vi "ReadGPS.vi"() -> ()   [LabVIEW 2010]
panel:
  in  "stop":bool
  out "GPS Data":T1 {"Course over ground (degrees)" format="%#.6g"; "Speed over ground (knots)" format="%#.6g"; "Magnetic Variation (degrees)" format="%#.6g"; "Longitude (ddmm.mmmm)" format="%#.6g"; "Lattitude (ddmm.mmmm)" format="%#.6g"}
  out "XY Graph":cluster{"Y":dbl[], "Y":dbl[]}[](graph)
  out "Course over ground (degrees)":dbl(knob) scale=0.0..360.0
  out "Speed over ground (knots)":dbl(knob) scale=0.0..5.0
  out "GPS Data Valid?":bool
  out "error out":errorcluster
  in  "VISA resource name":refnum<visa-resource-name>="COM1"
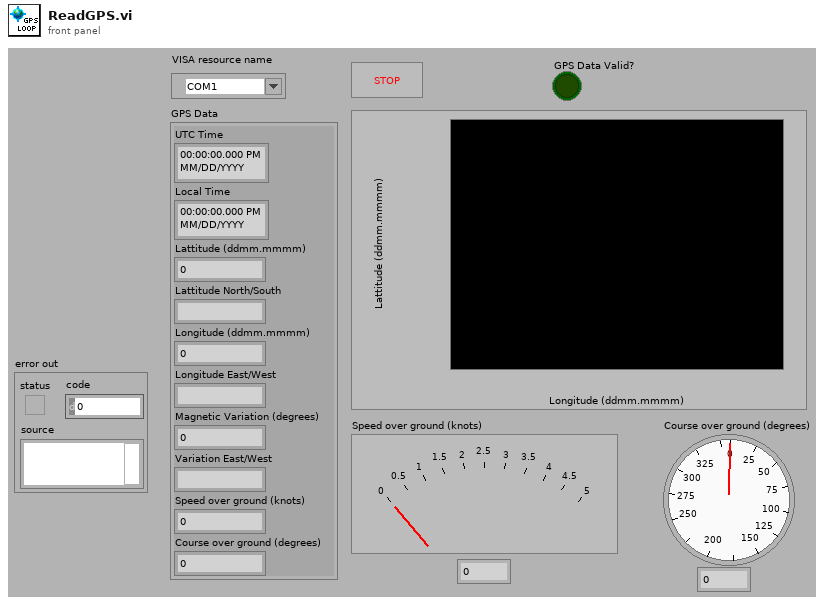
[diagram p1: front panel]
types:
  T1 = cluster{"UTC Time":timestamp, "Local Time":timestamp, "Lattitude (ddmm.mmmm)":dbl, "Lattitude North/South":string, "Longitude (ddmm.mmmm)":dbl, "Longitude East/West":string, "Magnetic Variation (degrees)":dbl, "Variation East/West":string, "Speed over ground (knots)":dbl, "Course over ground (degrees)":dbl}
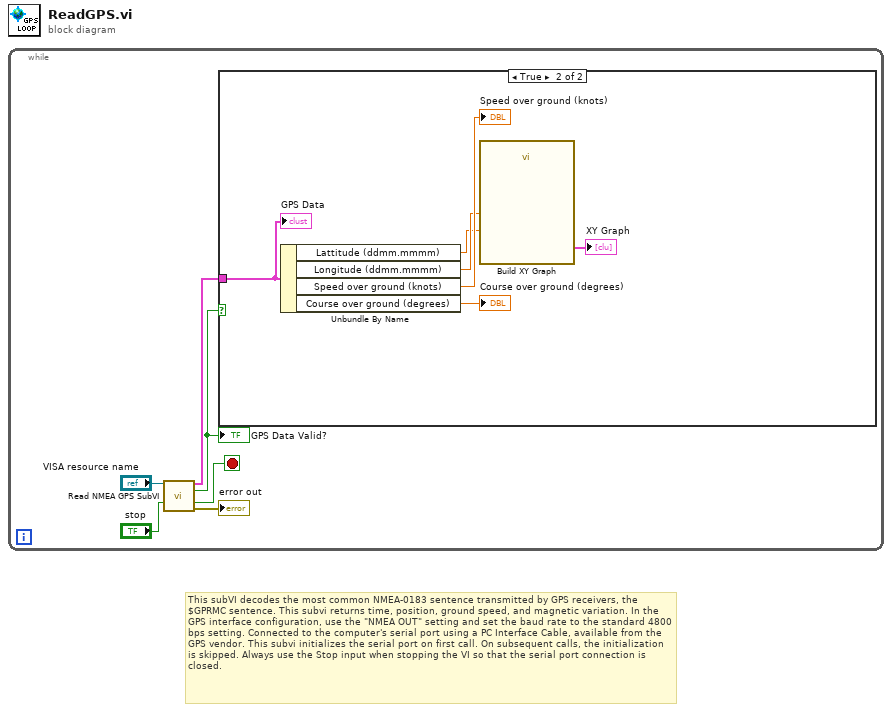
[diagram p0: block diagram]
diagram:
  # "This subVI decodes the most common NMEA-0183 sentence transmitted by GPS receivers, the $GPRMC sentence. This subvi returns time, position, ground speed, and magnetic variation. In the GPS interface configuration, use the \"NMEA OUT\" setting and set the baud rate to the standard 4800 bps setting. Connected to the computer's serial port using a PC Interface Cable, available from the GPS vendor. This subvi initializes the serial port on first call. On subsequent calls, the initialization is skipped. Always use the Stop input when stopping the VI so that the serial port connection is closed."
  n1 = while {
    stop <- w5 stop-if-true
    n2 = call "Read NMEA GPS SubVI.vi"("VISA resource name"="VISA resource name", "stop"="stop") -> ("GPS Data"=w3:T1, "GPS Data Valid?"=w4:bool, "Stopped?"=w5:bool, "error out"=→"error out":errorcluster)  [unwired: 10 in]
    "GPS Data Valid?" <- w4
    n3 = case shown="True" w4 {
      tunnel: w3 -> [_ w12]
      frame False {
      }
      frame True {
        n4 = Unbundle By Name(w12) -> ("Lattitude (ddmm.mmmm)"=w7:dbl, "Longitude (ddmm.mmmm)"=w8:dbl, "Speed over ground (knots)"=→"Speed over ground (knots)":dbl, "Course over ground (degrees)"=→"Course over ground (degrees)":dbl)
        n5 = call "Build XY Graph"("Y Input"=w7, "X Input"=w8) -> ("XY Graph"=→"XY Graph":cluster{"Y":dbl[], "Y":dbl[]}[])  [unwired: 8 in, 1 out]
        "GPS Data" <- w12
      }
    }
  }
